vi "dataconvert_array.vi"(8 "总时间（ms）":i32, 9 "相乘倍数":i32, 10 "每毫秒采样点":i32=1, 11 "输入的TTL信号序列":i32[](array[numeric])=[0, 0, 0, 0, 0, 0, 0, 0, 0, 0, 0, 0, 0, 0, 0, 0, 0, 0, 0, 0, 0, 0, 0, 0, 0, 0, 0, 0, 0, 0, 0, 0]) -> (2 "输出编码后的TTL序列":i32[](array[numeric]))   [LabVIEW 2021]
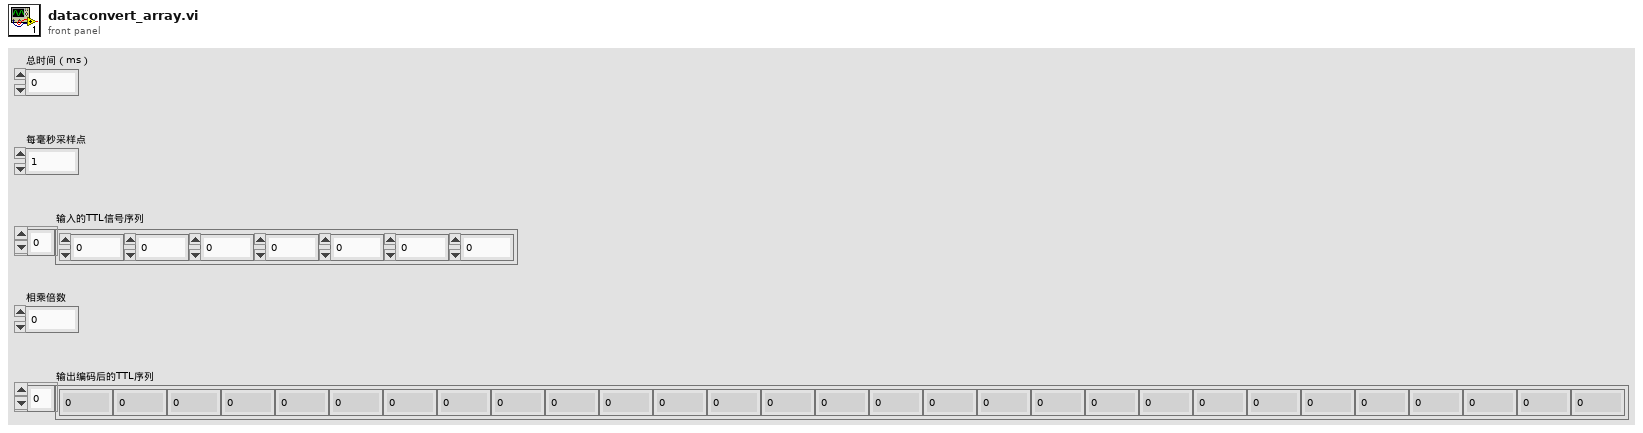
[diagram p1: front panel]
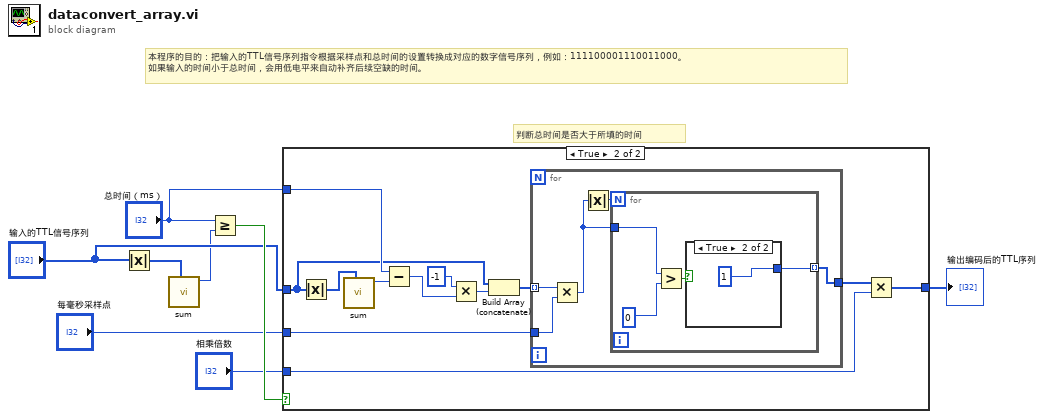
[diagram p0: block diagram]
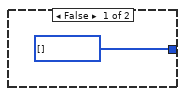
[diagram p2: hidden frame]
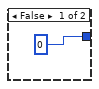
[diagram p3: hidden frame]
diagram:
  # "本程序的目的：把输入的TTL信号序列指令根据采样点和总时间的设置转换成对应的数字信号序列，例如：111100001110011000。\n如果输入的时间小于总时间，会用低电平来自动补齐后续空缺的时间。"
  # "判断总时间是否大于所填的时间"
  n1 = Absolute Value(x="输入的TTL信号序列") -> (abs(x)=w2:i32[])
  n2 = call "sum.vi"("numeric array"=w2) -> ("Numeric"=w3:i32)  [unwired: 9 in, 1 out]
  n3 = Greater Or Equal?(x="总时间（ms）", y=w3) -> (x >= y?=w8:bool)
  n4 = case shown="True" w8 {
    tunnel: "输入的TTL信号序列" -> [_ w18]
    tunnel: "每毫秒采样点" -> [_ w21]
    tunnel: "相乘倍数" -> [_ w20]
    tunnel: "总时间（ms）" -> [_ w19]
    tunnel: [i32[] [] w10] -> w1
    frame False {
    }
    frame True {
      n5 = Absolute Value(x=w18) -> (abs(x)=w11:i32[])
      n6 = call "sum.vi"("numeric array"=w11) -> ("Numeric"=w12:i32)  [unwired: 9 in, 1 out]
      n7 = Subtract(x=w19, y=w12) -> (x-y=w16:i32)
      n8 = Multiply(x=-1, y=w16) -> (x*y=w14:i32)
      n9 = Build Array (concatenate)(w18, w14) -> (w17:i32[])
      n10 = for {
        tunnel: w17 -> [w25] mode=indexing
        tunnel: w21 -> [w26]
        tunnel: [w22] -> w13
        n11 = Multiply(x=w25, y=w26) -> (x*y=w23:i32)
        n12 = Absolute Value(x=w23) -> (abs(x)=w24:i32)
        n13 = for {
          N: w24 -> [_]
          tunnel: w23 -> [w28]
          tunnel: [w27] -> w22 mode=indexing
          n14 = Greater?(x=w28, y=i16 0) -> (0:w30:bool)
          n15 = case shown="True" w30 {
            tunnel: [i16 0 i16 1] -> w27
            frame False {
            }
            frame True {
            }
          }
        }
      }
      n16 = Multiply(x=w13, y=w20) -> (x*y=w10:i32[])
    }
  }
  "输出编码后的TTL序列" <- w1
